vi "g_Panel Queue.vi"(6 "g_Panel Status(Get)":T1, 8 "error in (no error)":errorcluster, 9 "PanelName(\"\")":string, 11 "Queue":refnum<queue>) -> (0 "error out":errorcluster, 2 "Find?(False)":bool, 3 "Queue Out":refnum<queue>)   [LabVIEW 2015]
uses:
  Type Definition/g_Panel Status.ctl
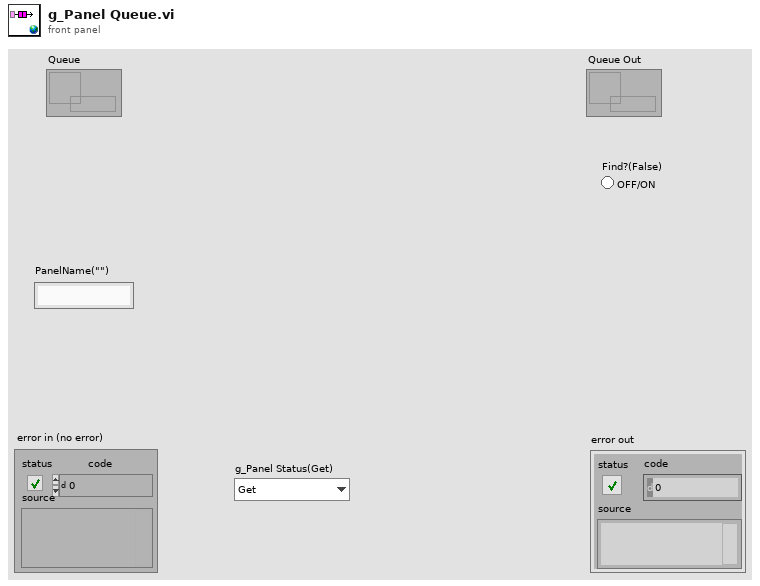
[diagram p1: front panel]
types:
  T1 = typedef "g_Panel Status.ctl" = enum16{"Get", "Set"}
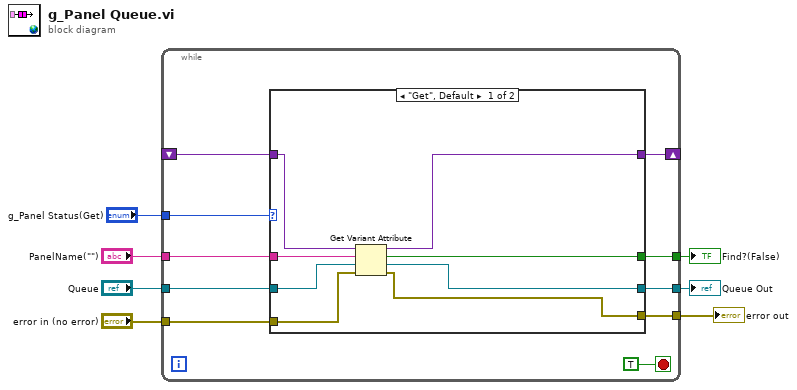
[diagram p0: block diagram]
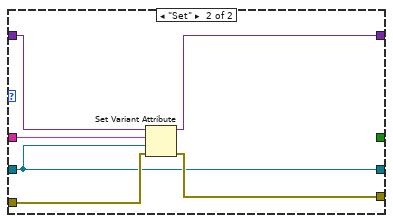
[diagram p2: hidden frame]
diagram:
  n1 = while {
    tunnel: "g_Panel Status(Get)" -> [w16]
    tunnel: "PanelName(\"\")" -> [w15]
    shift-right: [w10] -> _
    shift-left: _ -> [w14]
    tunnel: "Queue" -> [w13]
    tunnel: "error in (no error)" -> [w12]
    tunnel: [w11] -> w3
    tunnel: [w9] -> w2
    tunnel: [w8] -> w1
    stop <- TRUE stop-if-true
    n2 = case shown="\"Get\", Default" w16 {
      tunnel: w15 -> [w23 w30]
      tunnel: w14 -> [w25 w31]
      tunnel: w13 -> [w22 w26]
      tunnel: w12 -> [w24 w29]
      tunnel: [w19 w28] -> w11
      tunnel: [w20 w27] -> w10
      tunnel: [w21 w26] -> w9
      tunnel: [w18 _] -> w8
      frame "Get", Default {
        n3 = Get Variant Attribute(Variant=w25, name=w23, default value (empty Variant)=w22, error in=w24) -> (duplicate Variant=w20:variant, found=w18:bool, value=w21:refnum<queue>, error out=w19:errorcluster)
      }
      frame "Set" {
        n4 = Set Variant Attribute(Variant=w31, name=w30, value=w26, error in=w29) -> (Variant out=w27:variant, error out=w28:errorcluster)  [unwired: 1 out]
      }
    }
  }
  "error out" <- w3
  "Queue Out" <- w2
  "Find?(False)" <- w1
